vi "3D_Lab_v1.0.vi"() -> ()   [LabVIEW 2018]
uses:
  <vilib>/Native 3D Graph/xcontrol/3DPC_SurfacePlot.xctl
panel:
  out "3D Graph":refnum<class "Base Datatype.lvclass">[](xcontrol)
  out "X":dbl
  out "Z":dbl
  out "Y":dbl format="%#.8g"
  out "array":dbl[][](array[numeric])
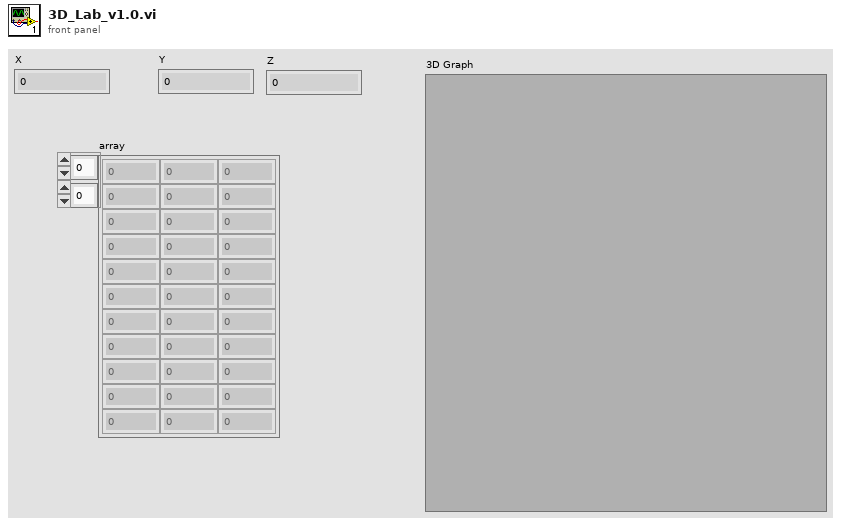
[diagram p1: front panel]
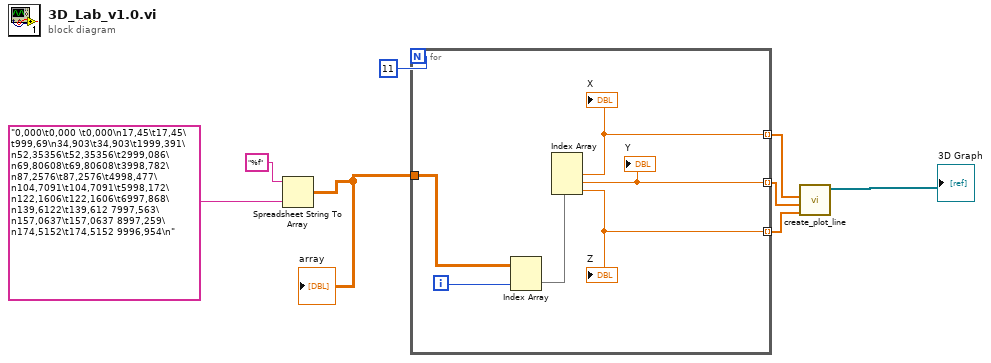
[diagram p0: block diagram]
diagram:
  n1 = Spreadsheet String To Array(format string="%f", spreadsheet string="0,000\t0,000 \t0,000\n17,45\t17,45\t999,69\n34,903\t34,903\t1999,391\n52,35356\t52,35356\t2999,086\n69,80608\t69,80608\t3998,782\n87,2576\t87,2576\t4998,477\n104,7091\t104,7091\t5998,172\n122,1606\t122,1606\t6997,868\n139,6122\t139,612 7997,563\n157,0637\t157,0637 8997,259\n174,5152\t174,5152 9996,954\n") -> (array=w6:dbl[][])  [unwired: 2 in]
  "array" <- w6
  n2 = for {
    N: 11 -> [_]
    tunnel: w6 -> [w12]
    tunnel: [w11] -> w1 mode=indexing
    tunnel: [w10] -> w2 mode=indexing
    tunnel: [w9] -> w3 mode=indexing
    i -> [w14]
    n3 = Index Array(array=w12, index (row)=w14) -> (element=w13:dbl[])  [unwired: 1 in]
    n4 = Index Array(array=w13) -> (element #1=w11:dbl, element #2=w10:dbl, element #3=w9:dbl)  [unwired: 3 in]
    "Y" <- w10
    "Z" <- w9
    "X" <- w11
  }
  n5 = call <vilib>:"create_plot_line.vi"("z vector"=w3, "y vector"=w2, "x vector"=w1) -> ("plots out"=→"3D Graph":refnum<class "Base Datatype.lvclass">[])  [unwired: 2 in, 6 out]
